vi "EvaluateEquation_v4.vi"(2 "Error Locator":string, 3 "error in (no error)":errorcluster, 4 "Current Variable settings":T1[](array[typedef]), 5 "formula":string) -> (0 "error out":errorcluster, 1 "y value":dbl)   [LabVIEW 2013]
doc: "The VI evaluates an expression using the LuaVIEW imbedded scripting language. A number of nice functions are defined (in the future it may well be better to define these via an initilizaion function).\n\nSome variables are predefined, but may be overwritten.\n\nt - in a ramp the total time elapsed since the start of the ramp\nf - in a ramp the fraction of the total time since the start of the ramp\ndt - in a ramp the time between timesteps\ntMax - in a ramp the total time"
uses:
  TypeDefs/Active procedure variables.ctl
  PackedLibraries/LuaEvaluatorAPI.lvlibp/API/t_Caching_Expression_Evaluator_Methods_Table.ctl
  PackedLibraries/LuaEvaluatorAPI.lvlibp
  Globals/UserFunctions.vi
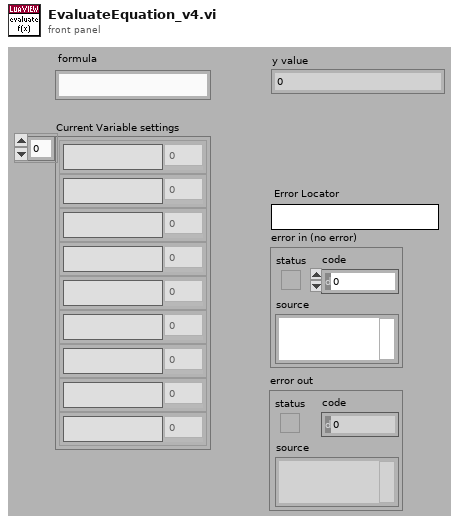
[diagram p1: front panel]
types:
  T1 = typedef "Active procedure variables.ctl" = cluster{"Procedure variable":string, "Value":dbl}
  T2 = typedef "LuaEvaluatorAPI.lvlibp/t_Caching_Expression_Evaluator_Methods_Table.ctl" = enum16{"set", "get", "eval", "assign", "isvalid", "execute", "evaltable", "close"}
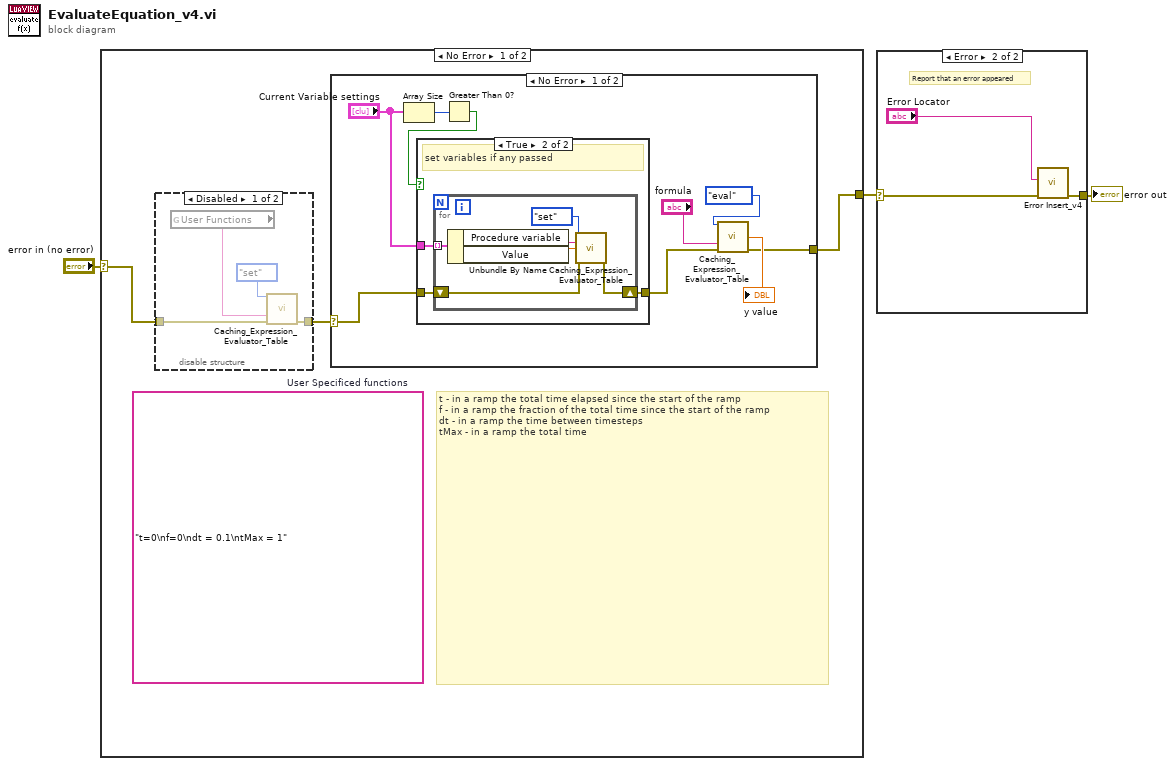
[diagram p0: block diagram]
diagram:
  n1 = case shown="No Error" "error in (no error)" {
    selector: "error in (no error)" -> [w4 w32]
    tunnel: [w6 w32] -> w2
    frame No Error {
      (unwired) "t=0\nf=0\ndt = 0.1\ntMax = 1"  # User Specificed functions
      # "t - in a ramp the total time elapsed since the start of the ramp\nf - in a ramp the fraction of the total time since the start of the ramp\ndt - in a ramp the time between timesteps\ntMax - in a ramp the total time"
      n2 = disable-structure shown="Disabled" {
        disable-tunnel: [w10 w11] -> w5
        disable-tunnel: w4 -> [w9 w11]
        frame Disabled {
          n3 = global read "UserFunctions.vi" "User Functions"() -> (w8:string)
          n4 = call "Caching_Expression_Evaluator_Table.vi"("method"=t_Caching_Expression_Evaluator_Methods_Table."set", "expression/scriptlet"=w8, "error in (no error)"=w9) -> ("error out"=w10:errorcluster)  [unwired: 4 in, 8 out]
        }
        frame Enabled {
        }
      }
      n5 = case shown="No Error" w5 {
        selector: w5 -> [w17 w31]
        tunnel: [w16 w31] -> w6
        frame No Error {
          n6 = Array Size(array="Current Variable settings") -> (size(s)=w14:i32)
          n7 = Greater Than 0?(x=w14) -> (x > 0?=w13:bool)
          n8 = case shown="True" w13 {
            tunnel: [w21 w24] -> w20
            tunnel: w17 -> [w21 w23]
            tunnel: "Current Variable settings" -> [_ w22]
            frame False {
              # "Lua remembers all set variables so there is no need to re-set them on each evaluate call!"
              # "no varibales passed"
            }
            frame True {
              # "set variables if any passed"
              n9 = for {
                shift-right: [w30] -> w24
                shift-left: w23 -> [w29]
                tunnel: w22 -> [w28] mode=indexing
                n10 = Unbundle By Name(w28) -> ("Procedure variable"=w27:string, "Value"=w26:dbl)
                n11 = call "Caching_Expression_Evaluator_Table.vi"("method"=t_Caching_Expression_Evaluator_Methods_Table."set", "variable"=w27, "value in"=w26, "error in (no error)"=w29) -> ("error out"=w30:errorcluster)  [unwired: 9 in, 2 out]
              }
            }
          }
          n12 = call "Caching_Expression_Evaluator_Table.vi"("method"=t_Caching_Expression_Evaluator_Methods_Table."eval", "expression/scriptlet"="formula", "error in (no error)"=w20) -> ("value out"=→"y value":dbl, "error out"=w16:errorcluster)  [unwired: 10 in, 1 out]
        }
        frame Error {
        }
      }
    }
    frame Error {
    }
  }
  n13 = case shown="Error" w2 {
    selector: w2 -> [w33 w36]
    tunnel: [w33 w35] -> w1
    frame No Error {
    }
    frame Error {
      # "Report that an error appeared"
      n14 = call "Error Insert_v4.vi"("error in (no error)"=w36, "error message (\"\")"="Error Locator") -> ("error out"=w35:errorcluster)  [unwired: 1 in, 6 out]
    }
  }
  "error out" <- w1
